vi "EncodeImageFileToBase64.vi"(8 "error in (no error)":errorcluster, 11 "ImagePath":path) -> (0 "error out":errorcluster, 3 "Base64String":string)   [LabVIEW 2020]
doc: "Encode an image file to a Base64 Data URI"
uses:
  <vilib>/Utility/error.llb/Error Cluster From Error Code.vi
  <vilib>/ErrorRing/Error Ring.xnode
  <vilib>/JDP Science/JDP Science Common Utilities/Base64/Base64 Support.lvlib
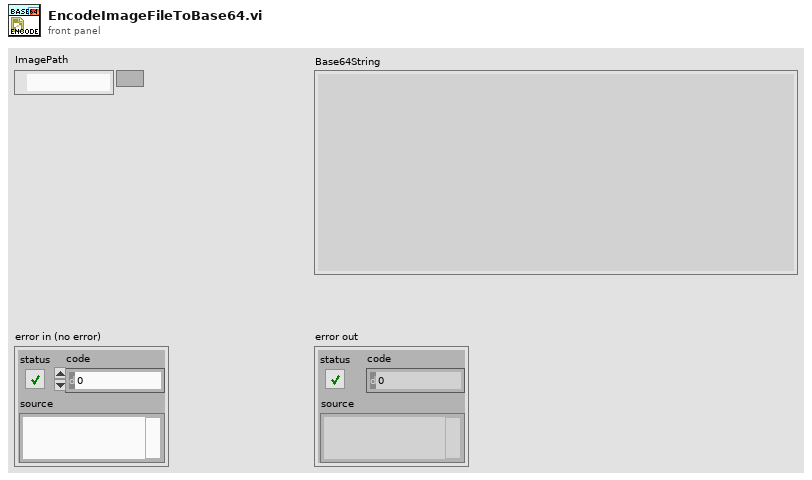
[diagram p1: front panel]
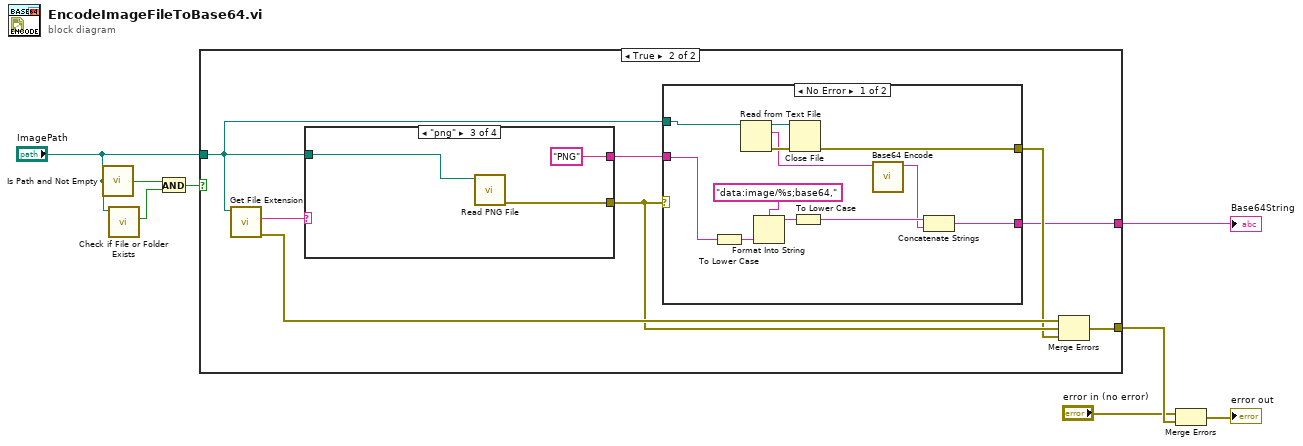
[diagram p0: block diagram]
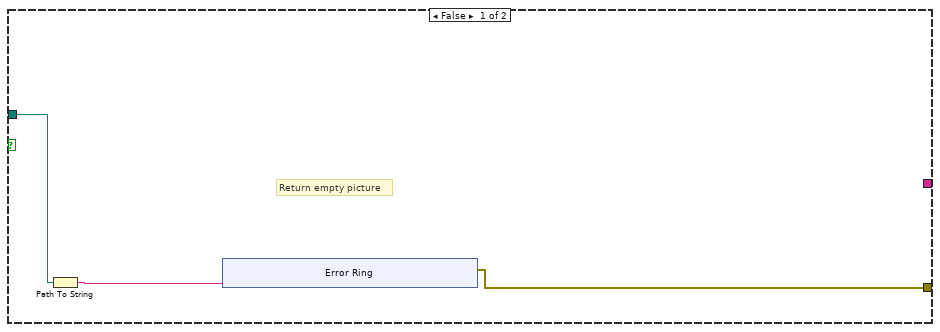
[diagram p2: hidden frame]
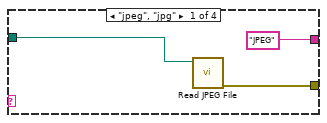
[diagram p4: hidden frame]
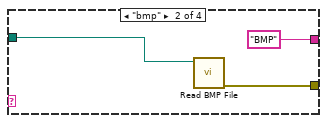
[diagram p5: hidden frame]
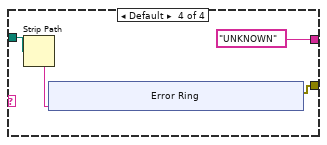
[diagram p6: hidden frame]
diagram:
  n1 = call <vilib>:"Is Path and Not Empty.vi"("path"="ImagePath") -> ("Is Path and Not Empty?"=w7:bool)  [unwired: 4 in]
  n2 = call <vilib>:"Check if File or Folder Exists.vi"("path"="ImagePath") -> ("file or folder exists?"=w8:bool)  [unwired: 8 in, 2 out]
  n3 = And(x=w7, y=w8) -> (x .and. y?=w1:bool)
  n4 = case shown="True" w1 {
    tunnel: "ImagePath" -> [w10 w21]
    tunnel: [w9 w24] -> w5
    tunnel: [_ w19] -> w2
    frame False {
      # "Return empty picture"
      n5 = Path To String(path=w10) -> (string=w11:string)
      n6 = xnode "Error Ring"("parameter 0"=w11) -> ("error out"=w9:errorcluster)
    }
    frame True {
      n7 = call <vilib>:"Get File Extension.vi"("file"=w21) -> ("error out"=w25:errorcluster, "lowercase file extension"=w26:string)  [unwired: 6 in, 3 out]
      n8 = case shown="\"png\"" w26 {
        tunnel: w21 -> [w41 w43 w46 w50]
        tunnel: [w40 w44 w47 w51] -> w22
        tunnel: ["JPEG" "BMP" "PNG" "UNKNOWN"] -> w23
        frame "jpeg", "jpg" {
          n9 = call <vilib>:"Read JPEG File.vi"("path to JPEG file"=w41) -> ("error out"=w40:errorcluster)  [unwired: 8 in, 2 out]
        }
        frame "bmp" {
          n10 = call <vilib>:"Read BMP File.vi"("path to BMP file"=w43) -> ("error out"=w44:errorcluster)  [unwired: 8 in, 2 out]
        }
        frame "png" {
          n11 = call <vilib>:"Read PNG File.vi"("path to PNG file"=w46) -> ("error out"=w47:errorcluster)  [unwired: 8 in, 2 out]
        }
        frame Default {
          n12 = Strip Path(path=w50) -> (name=w49:string)  [unwired: 1 out]
          n13 = xnode "Error Ring"("parameter 0"=w49) -> ("error out"=w51:errorcluster)
        }
      }
      n14 = case shown="No Error" w22 {
        tunnel: w23 -> [w37 _]
        tunnel: w21 -> [w36 _]
        tunnel: [w29 _] -> w20
        tunnel: [w28 _] -> w19
        frame No Error {
          n15 = To Lower Case(string=w37) -> (all lower case string=w27:string)
          n16 = Read from Text File(file (use dialog)=w36) -> (refnum out=w34:refnum<file>, text=w33:string, error out=w35:errorcluster)  [unwired: 3 in, 1 out]
          n17 = Format Into String(format string="data:image/%s;base64,", w27) -> (resulting string=w38:string)  [unwired: 2 in, 1 out]
          n18 = Close File(refnum=w34, error in=w35) -> (error out=w29:errorcluster)  [unwired: 1 out]
          n19 = To Lower Case(string=w38) -> (all lower case string=w31:string)
          n20 = call <vilib>:"Base64 Encode.vi"("String to Encode"=w33) -> ("Base64 Encoded"=w30:string)  [unwired: 10 in]
          n21 = Concatenate Strings(w31, w30) -> (w28:string)
        }
        frame Error {
        }
      }
      n22 = Merge Errors(w25, w22, w20) -> (w24:errorcluster)
    }
  }
  "Base64String" <- w2
  n23 = Merge Errors("error in (no error)", w5) -> (→"error out":errorcluster)
